vi "File_Module.vi"(7 "Command":T2, 8 "error in (no error)":errorcluster, 9 "DATOS":T1={"TIEMPO"=1.0, "SET_TH"=1.0, "TEMP_TH"=1.0, "SET_TC"=0.0, "TEMP_TC"=0.0, "eVAL_5"=0.0, "a FSET1"=0.0, "a FLUJO1"=0.0, "a FSET2"=0.0, "a FLUJO2"=0.0, "a FSET3"=0.0, "a FLUJO3"=0.0, "a FSET4"=0.0, "a FLUJO4"=0.0} {"a FSET4" format="%.2g"; "a FSET3" format="%.2g"; "a FSET2" format="%.2g"; "a FSET1" format="%.2g"; "a FLUJO4" format="%.2g"; "a FLUJO2" format="%.2g"; "a FLUJO1" format="%.2g"; "a FLUJO3" format="%.2g"; "eVAL_5" format="%.2g"; "TEMP_TH" format="%.2g"; "SET_TH" format="%.2g"; "TEMP_TC" format="%.2g"; "SET_TC" format="%.2g"; "TIEMPO" format="%.2g"}, 11 "Comments":string) -> (0 "error out":errorcluster, 2 "selected path":path)   [LabVIEW 2017]
uses:
  File_Module Control.ctl
  REACTOR_DATOS.ctl
  REACTOR_GLOBALES.vi
panel:
  out "Cabeceras":string[](array[string])
  # "COMENTARIOS NO ACTUALIZADOS"
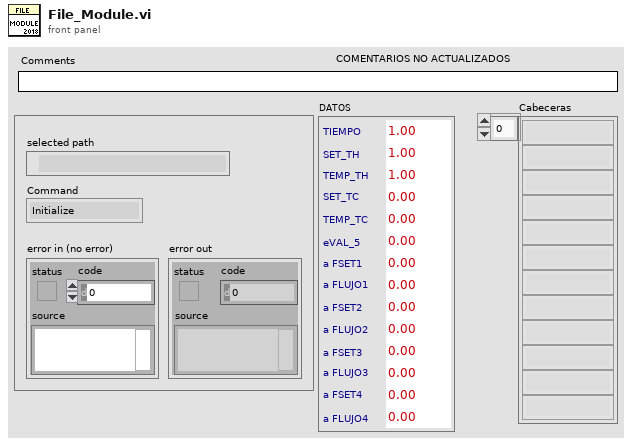
[diagram p1: front panel]
types:
  T1 = typedef "REACTOR_DATOS.ctl" = cluster{"TIEMPO":dbl, "SET_TH":dbl, "TEMP_TH":dbl, "SET_TC":dbl, "TEMP_TC":dbl, "eVAL_5":dbl, "a FSET1":dbl, "a FLUJO1":dbl, "a FSET2":dbl, "a FLUJO2":dbl, "a FSET3":dbl, "a FLUJO3":dbl, "a FSET4":dbl, "a FLUJO4":dbl}
  T2 = typedef "File_Module Control.ctl" = enum16{"Initialize", "Save Head", "Save Data", "Shutdown"}
  T3 = enum16{"open", "replace", "create", "open or create", "replace or create", "replace or create with confirmation"}
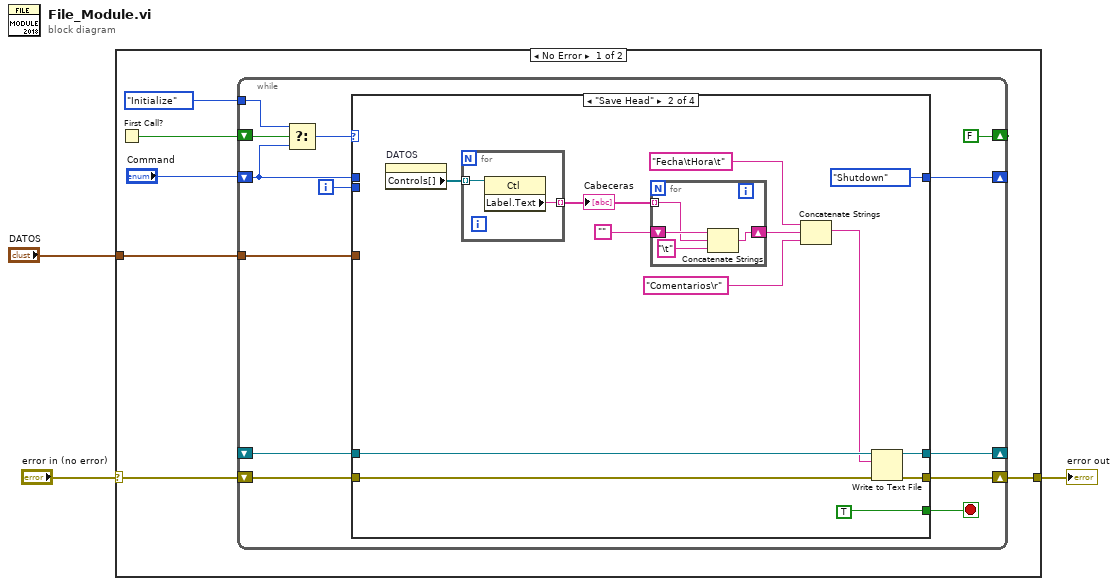
[diagram p0: block diagram]
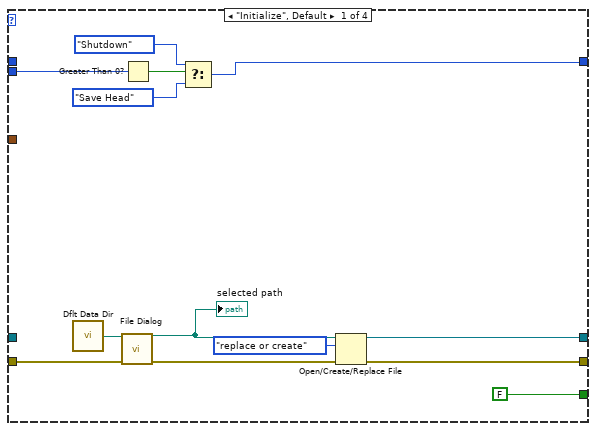
[diagram p2: hidden frame]
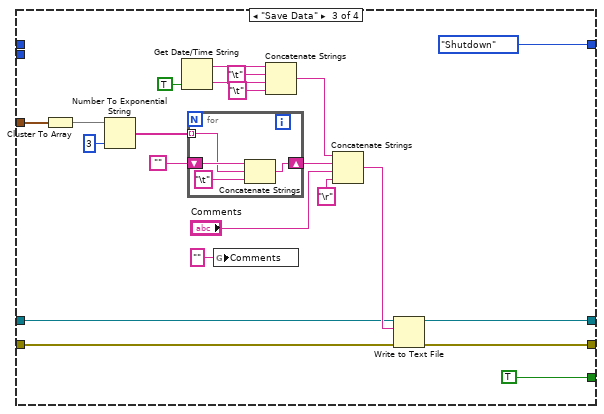
[diagram p3: hidden frame]
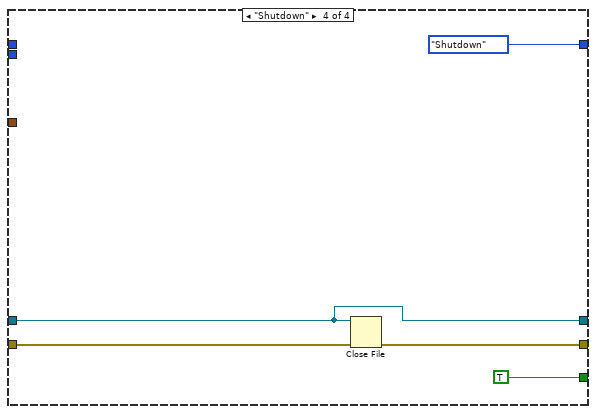
[diagram p4: hidden frame]
diagram:
  n1 = case shown="No Error" "error in (no error)" {
    selector: "error in (no error)" -> [w7 w86]
    tunnel: [w6 w86] -> w2
    tunnel: "DATOS" -> [w4 _]
    frame No Error {
      n2 = First Call?() -> (First Call?: T/F=w9:bool)
      n3 = while {
        shift-right: [w14] -> _
        shift-left: "Command" -> [w15]
        shift-right: [w17] -> w6
        shift-left: w7 -> [w18]
        shift-right: [FALSE ("First Call?: T/F")] -> _
        shift-left: w9 -> [w22]
        tunnel: File_Module_Control."Initialize" ("t") -> [w21]
        shift-right: [w11] -> _
        shift-left: _ -> [w12]
        tunnel: w4 -> [w10]
        i -> [w13]
        stop <- w19 stop-if-true
        n4 = Select(t=w21, s=w22, f=w15) -> (s? t:f=w20:T2)
        n5 = case shown="\"Save Head\"" w20 {
          tunnel: [FALSE TRUE TRUE TRUE] -> w19
          tunnel: w18 -> [w28 w44 w68 w83]
          tunnel: [w24 w43 w67 w82] -> w17
          tunnel: w15 -> [_ _ _ _]
          tunnel: [w34 File_Module_Control."Shutdown" ("t") File_Module_Control."Shutdown" File_Module_Control."Shutdown"] -> w14
          tunnel: w13 -> [w32 _ _ _]
          tunnel: w12 -> [_ w46 w64 w81]
          tunnel: [w23 w45 w66 w81] -> w11
          tunnel: w10 -> [_ _ w70 _]
          frame "Initialize", Default {
            n6 = call <vilib>:"Dflt Data Dir.vi"() -> ("App:Default Data Directory"=w29:path)
            n7 = call "File Dialog"("start path"=w29, "error in"=w28) -> ("selected path"=w26:path, "error out"=w25:errorcluster)  [unwired: 10 in, 2 out]
            "selected path" <- w26
            n8 = Greater Than 0?(x=w32) -> (x > 0?=w31:bool)
            n9 = Select(t=File_Module_Control."Shutdown", s=w31, f=File_Module_Control."Save Head" ("t")) -> (s? t:f=w34:T2)
            n10 = Open/Create/Replace File(file path (use dialog)=w26, error in=w25, operation (0:open)=T3."replace or create") -> (refnum out=w23:refnum<file>, error out=w24:errorcluster)  [unwired: 3 in, 1 out]
          }
          frame "Save Head" {
            n11 = property on="DATOS" class="Clust (strict)"() -> ("Controls[]"=w42:refnum<vi>[])  [unwired: 2 in, 2 out]
            n12 = for {
              tunnel: w42 -> [w54] mode=indexing
              tunnel: [w53] -> w38 mode=indexing
              n13 = property class="Ctl"(reference=w54) -> ("Label.Text"=w53:string)  [unwired: 1 in, 2 out]
            }
            "Cabeceras" <- w38
            n14 = for {
              tunnel: w38 -> [w51] mode=indexing
              shift-right: [w50] -> w41
              shift-left: "" -> [w52]
              n15 = Concatenate Strings(w52, w51, "\t" ("string")) -> (w50:string)
            }
            n16 = Concatenate Strings("Fecha\tHora\t" ("string"), w41, "Comentarios\r" ("string")) -> (w36:string)
            n17 = Write to Text File(file (use dialog)=w46, text=w36, error in=w44) -> (refnum out=w45:refnum<file>, error out=w43:errorcluster)  [unwired: 1 in, 1 out]
          }
          frame "Save Data" {
            n18 = Cluster To Array(cluster=w70) -> (array=w71:dbl[])
            n19 = Number To Exponential String(number=w71, precision (6)=i16 3) -> (E-format string=w69:string[])  [unwired: 2 in]
            n20 = Get Date/Time String(want seconds? (F)=TRUE) -> (date string=w60:string, time string=w59:string)  [unwired: 2 in]
            n21 = for {
              tunnel: w69 -> [w79] mode=indexing
              shift-right: [w78] -> w74
              shift-left: "" -> [w80]
              n22 = Concatenate Strings(w80, w79, "\t" ("string")) -> (w78:string)
            }
            n23 = global write "REACTOR_GLOBALES.vi" "Comments"("" ("Comments")) -> ()
            n24 = Concatenate Strings(w60, "\t" ("string"), w59, "\t" ("string")) -> (w63:string)
            n25 = Concatenate Strings(w63, w74, "Comments", "\r" ("string")) -> (w65:string)
            n26 = Write to Text File(file (use dialog)=w64, text=w65, error in=w68) -> (refnum out=w66:refnum<file>, error out=w67:errorcluster)  [unwired: 1 in, 1 out]
          }
          frame "Shutdown" {
            n27 = Close File(refnum=w81, error in=w83) -> (error out=w82:errorcluster)  [unwired: 1 out]
          }
        }
      }
    }
    frame Error {
    }
  }
  "error out" <- w2
